vi "Test MFC ESF.vi"() -> ()   [LabVIEW 2014, in "Alicat Lib.lvlib" / "Alicat Device.lvclass"]
uses:
  Alicat Device.lvclass
  reusable/Session APIs/File Access/Config Data/Config Session.ctl
  reusable/Session APIs/File Access/Config Data/Config Data.lvclass
  reusable/Session APIs/File Access/Config Data/Config Data.lvclass/Config Data.ctl
  Configurable Device/Configurable Device.lvclass/Configurable Device.ctl
  Data/MC/MC Data.lvclass
  Data/M/M data.lvclass
  Data/MC/MC Data.lvclass/MC Data.ctl
  Data/M/M data.lvclass/M data.ctl
  reusable/Session APIs/Serial/Serial Session.lvclass
  Alicat Device.lvclass/Alicat Device.ctl
  Configurable Device/Write Handle.vi
  Configurable Device/Write ID.vi
  Data/MC/Accessors/Read P.vi
  Data/MC/Accessors/Read T.vi
  Data/M/Accessors/Read P.vi
  Data/M/Accessors/Read T.vi
  reusable/Session APIs/File Access/Config Data/Accessors/Write Cfg Path.vi
  reusable/Data/Read measTime.vi
  <userlib>/_Session Fwk/Session - Root.lvclass
panel:
  out "Time":timestamp[](array[timestamp]) format="%<%H:%M:%S%2u>T"
  out "dataOut":cluster{"Accessors:P":sgl, "Accessors:T":sgl}[](graph) caption="Alicat Data"
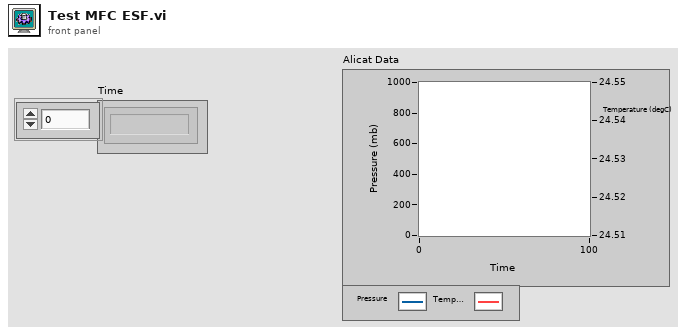
[diagram p1: front panel]
types:
  T1 = typedef "Config Data.lvclass/Config Session.ctl" = refnum<data-value>
  T2 = typedef "Session - Root.lvclass/Session Handle.ctl" = refnum<data-value>
  T3 = typedef "Serial Session.lvclass/Session Handle.ctl" = refnum<data-value>
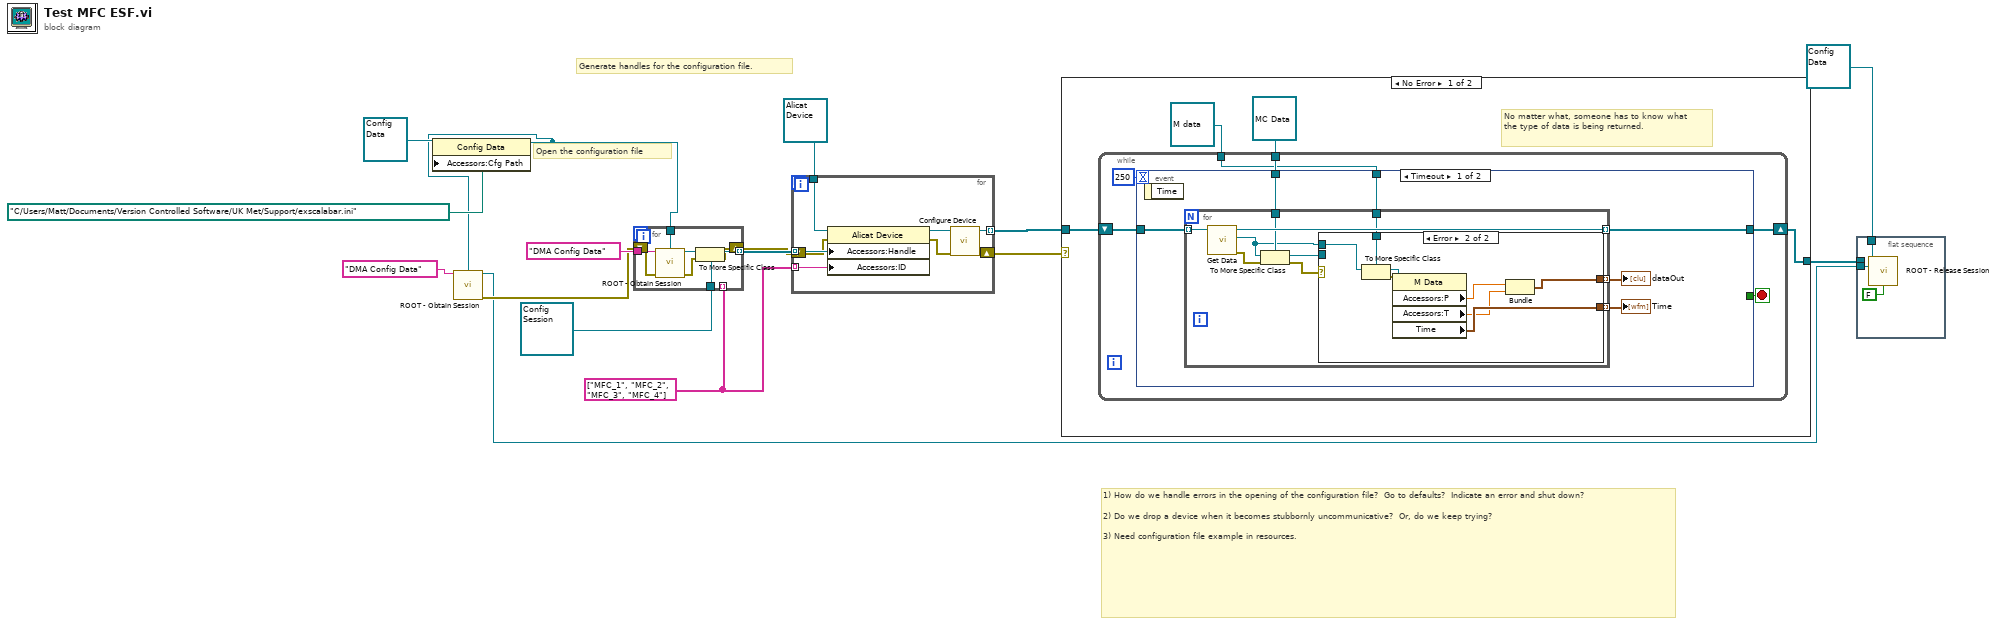
[diagram p0: block diagram]
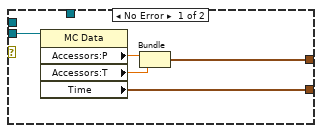
[diagram p2: hidden frame]
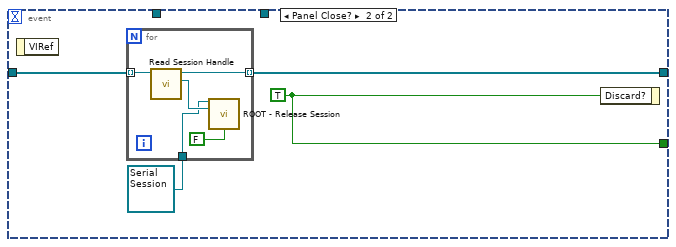
[diagram p3: hidden frame]
diagram:
  w12 = string[] ["MFC_1", "MFC_2", "MFC_3", "MFC_4"]
  # "1) How do we handle errors in the opening of the configuration file?  Go to defaults?  Indicate an error and shut down?\n\n2) Do we drop a device when it becomes stubbornly uncommunicative?  Or, do we keep trying?\n\n3) Need configuration file example in resources."
  # "Open the configuration file"
  # "Generate handles for the configuration file."
  n1 = property class="Config Data"(reference=refnum<class "Config Data.lvclass"> refnum ("Config Data"), "Accessors:Cfg Path"=path "C:/Users/Matt/Documents/Version Controlled Software/UK Met/Support/exscalabar.ini" ("Path")) -> (reference out=w6:refnum<class "Config Data.lvclass">)  [unwired: 1 in, 1 out]
  n2 = call <userlib>:"ROOT - Obtain Session.vi"("Session Name ()"="DMA Config Data", "OBJ - Session"=w6) -> ("Session Handle"=w2:T2, "error out"=w5:errorcluster)  [unwired: 11 in, 1 out]
  n3 = for {
    tunnel: w6 -> [w23]
    tunnel: T1 refnum ("Session Handle") -> [w22]
    tunnel: [w21] -> w13 mode=indexing
    tunnel: w12 -> [_] mode=indexing
    tunnel: "DMA Config Data" ("Session Name ()") -> [w20]
    shift-right: [w18] -> w8
    shift-left: w5 -> [w17]
    n4 = call <userlib>:"ROOT - Obtain Session.vi"("Session Name ()"=w20, "OBJ - Session"=w23, "error in (no error)"=w17) -> ("Session Handle"=w24:T2, "error out"=w19:errorcluster)  [unwired: 10 in, 1 out]
    n5 = To More Specific Class(target class=w22, reference=w24, error in=w19) -> (specific class reference=w21:T1, error out=w18:errorcluster)
  }
  n6 = for {
    tunnel: w12 -> [w30] mode=indexing
    tunnel: [w32] -> w16 mode=indexing
    tunnel: refnum<class "Alicat Device.lvclass"> refnum ("Alicat Device in") -> [w31]
    tunnel: w13 -> [w27] mode=indexing
    shift-right: [w25] -> w1
    shift-left: w8 -> [w26]
    n7 = property class="Alicat Device"(reference=w31, error in=w26, "Accessors:Handle"=w27, "Accessors:ID"=w30) -> (reference out=w29:refnum<class "Alicat Device.lvclass">, error out=w28:errorcluster)
    n8 = call-dynamic "Configure Device.vi"("error in"=w28, "Alicat Device In"=w29) -> ("error out"=w25:errorcluster, "Alicat Device Out"=w32:refnum<class "Alicat Device.lvclass">)  [unwired: 5 in, 3 out]
  }
  n9 = case shown="No Error" w1 {
    tunnel: w16 -> [w35 _]
    tunnel: [w33 _] -> w4
    frame No Error {
      # "No matter what, someone has to know what the type of data is being returned."
      n10 = while {
        shift-right: [w39] -> w33
        shift-left: w35 -> [w41]
        tunnel: refnum<class "MC Data.lvclass"> refnum ("MC Data") -> [w38]
        tunnel: refnum<class "M data.lvclass"> refnum ("M Data") -> [w37]
        stop <- w42 stop-if-true
        n11 = event shown="[0] Timeout" {
          selector: _ -> [_ _]
          dyn-events: _ -> [_ _]
          timeout: 250 -> [_ _]
          tunnel: [_ w75] -> w42
          tunnel: w41 -> [w46 w73]
          tunnel: [w48 w74] -> w39
          tunnel: w38 -> [w47 _]
          tunnel: w37 -> [w43 _]
          event Timeout {
            n12 = event-data() -> ()  [unwired: 1 in, 1 out]
            n13 = for {
              tunnel: [w58] -> w48 mode=indexing
              tunnel: w47 -> [w56]
              tunnel: w46 -> [w54] mode=indexing
              tunnel: [w53] -> w45 mode=indexing
              tunnel: [w52] -> w44 mode=indexing
              tunnel: w43 -> [w50]
              n14 = call-dynamic "Get Data.vi"("Alicat Device in"=w54) -> ("error out"=w57:errorcluster, "Data"=w49:refnum<class "Data.lvclass">, "Alicat Device out"=w58:refnum<class "Alicat Device.lvclass">)  [unwired: 8 in]
              n15 = To More Specific Class(target class=w56, reference=w49, error in=w57) -> (specific class reference=w55:refnum<class "MC Data.lvclass">, error out=w51:errorcluster)
              n16 = case shown="Error" w51 {
                tunnel: w55 -> [w63 _]
                tunnel: [w60 w64] -> w53
                tunnel: [w59 w67] -> w52
                tunnel: w49 -> [_ w71]
                tunnel: w50 -> [_ w70]
                frame No Error {
                  n17 = property class="MC Data"(reference=w63) -> ("Accessors:P"=w62:sgl, "Accessors:T"=w61:sgl, "Time"=w59:timestamp)  [unwired: 1 in, 2 out]
                  n18 = Bundle("Accessors:P"=w62, "Accessors:T"=w61) -> (w60:cluster{"Accessors:P":sgl, "Accessors:T":sgl})  [unwired: 1 in]
                }
                frame Error {
                  n19 = To More Specific Class(target class=w70, reference=w71) -> (specific class reference=w68:refnum<class "M data.lvclass">, error out=w69:errorcluster)  [unwired: 1 in]
                  n20 = property class="M Data"(reference=w68, error in=w69) -> ("Accessors:P"=w66:sgl, "Accessors:T"=w65:sgl, "Time"=w67:timestamp)  [unwired: 2 out]
                  n21 = Bundle("Accessors:P"=w66, "Accessors:T"=w65) -> (w64:cluster{"Accessors:P":sgl, "Accessors:T":sgl})  [unwired: 1 in]
                }
              }
            }
            "dataOut" <- w45
            "Time" <- w44
          }
          event Panel Close? {
            w75 = TRUE ("Discard?")
            n22 = event-data() -> ()  [unwired: 1 in, 1 out]
            n23 = for {
              tunnel: [w80] -> w74 mode=indexing
              tunnel: w73 -> [w79] mode=indexing
              tunnel: refnum<class "Serial Session.lvclass"> refnum ("Serial Session") -> [w76]
              n24 = call "Read Session Handle.vi"("Alicat Device in"=w79) -> ("Session Handle"=w78:T3, "Alicat Device out"=w80:refnum<class "Alicat Device.lvclass">)  [unwired: 8 in, 1 out]
              n25 = call <userlib>:"ROOT - Release Session.vi"("OBJ - Session in"=w76, "Session Handle in"=w78, "force destroy? (F)"=FALSE) -> ()  [unwired: 11 in, 2 out]
            }
            n26 = event-data("Discard?"=w75) -> ()  [unwired: 1 in, 1 out]
          }
        }
      }
    }
    frame Error {
    }
  }
  n27 = flat-sequence {
    tunnel: w4 -> [_]
    tunnel: refnum<class "Config Data.lvclass"> refnum ("Config Data") -> [w83]
    tunnel: w2 -> [w82]
    frame #0 {
      n28 = call <userlib>:"ROOT - Release Session.vi"("OBJ - Session in"=w83, "Session Handle in"=w82, "force destroy? (F)"=FALSE) -> ()  [unwired: 11 in, 2 out]
    }
  }
